vi "Lab02_LabViewArray&ForLoopP1_Bennett.vi"() -> ()   [LabVIEW 2017]
uses:
  <vilib>/Analysis/baseanly.llb/Mean (DBL).vi
  <vilib>/Analysis/NI_AALBase.lvlib
panel:
  out "Mean (By LV)":dbl
  out "Mean (By Calc)":dbl
  in  "Num List":dbl[](array[numeric])
  # "ELEC3800: IoT                      Lab02: Part I                      Matt Bennett\nFall 2017                                                                           09/12/17"
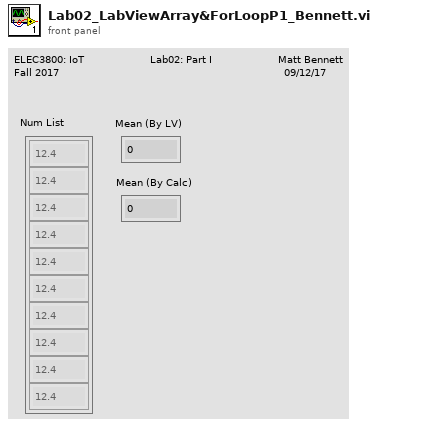
[diagram p1: front panel]
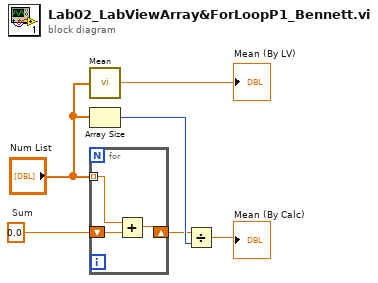
[diagram p0: block diagram]
diagram:
  w6 = 0.0  # Sum
  n1 = call-poly <vilib>:"Mean.vi"("X"="Num List") -> ("mean"=→"Mean (By LV)":dbl)  [unwired: 1 out]
  n2 = Array Size(array="Num List") -> (size(s)=w5:i32)
  n3 = for {
    tunnel: "Num List" -> [w9] mode=indexing
    shift-right: [w7] -> w4
    shift-left: w6 -> [w8]
    n4 = Add(x=w9, y=w8) -> (x+y=w7:dbl)
  }
  n5 = Divide(x=w4, y=w5) -> (x/y=→"Mean (By Calc)":dbl)
